vi "Fetch Waveform.vi"(8 "error in (no error)":errorcluster, 9 "Timeout (10000 ms)":u32=10000, 10 "Channel (1: Channel 1)":u16(ring)=1 items=["Channel 1"=1, "Channel 2"=2, "Channel 3"=3, "Channel 4"=4], 11 "VISA resource name":refnum<visa-resource-name>) -> (0 "error out":errorcluster, 2 "Waveform Data":waveform(dbl)(graph), 3 "VISA resource name out":refnum<visa-resource-name>)   [LabVIEW 2023, in "RIGOL DS1054Z Driver.lvlib"]
doc: "Returns the waveform the oscilloscope acquired for the specified channel. The waveform is from an acquisition that you initiate prior to calling this VI.\n\n<B>Note:</B>\n Use this VI only with other low-level VIs."
uses:
  <instrlib>/RIGOL-DS1054Z-LabVIEW/RIGOL DS1054Z Driver.lvlib
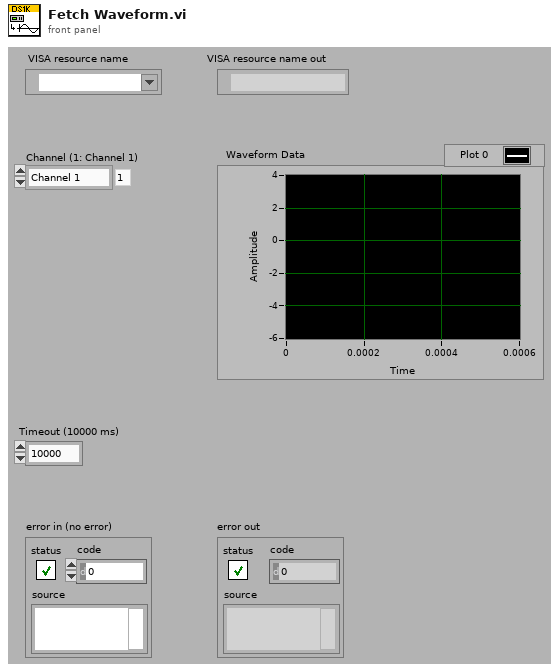
[diagram p1: front panel]
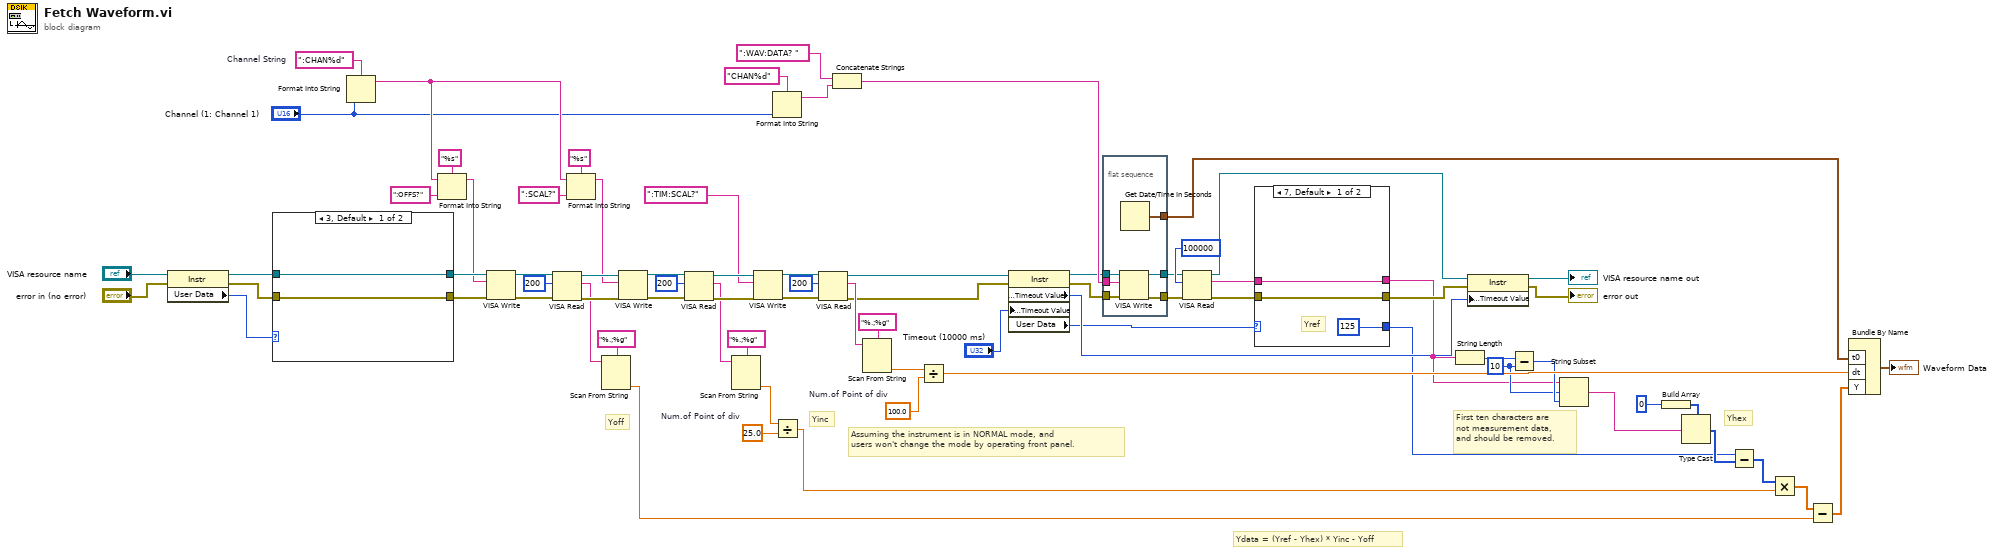
[diagram p0: block diagram]
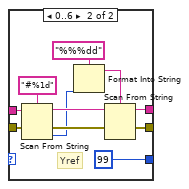
[diagram p2: hidden frame]
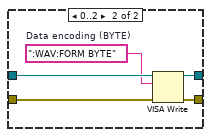
[diagram p3: hidden frame]
diagram:
  w6 = ":CHAN%d"  # Channel String
  w9 = 10 ("y")
  w21 = 100.0  # Num.of Point of div
  w30 = 25.0  # Num.of Point of div
  # "Assuming the instrument is in NORMAL mode, and \nusers won't change the mode by operating front panel."
  # "First ten characters are\nnot measurement data, \nand should be removed."
  # "Yoff"
  # "Yinc"
  # "Yhex"
  # "Ydata = (Yref - Yhex) * Yinc - Yoff"
  n1 = property class="Instr"(reference="VISA resource name", error in="error in (no error)") -> (reference out=w60:refnum<visa-resource-name>, error out=w58:errorcluster, "User Data"=w39:u32)
  n2 = case shown="3, Default" w39 {
    tunnel: [w79 w84] -> w57
    tunnel: [w78 w83] -> w56
    tunnel: w60 -> [w79 w82]
    tunnel: w58 -> [w78 w81]
    frame 3, Default {
    }
    frame 0..2 {
      w80 = ":WAV:FORM BYTE"  # Data encoding (BYTE)
      n3 = VISA Write(VISA resource name=w82, write buffer=w80, error in (no error)=w81) -> (VISA resource name out=w84:refnum<visa-resource-name>, error out=w83:errorcluster)  [unwired: 1 out]
    }
  }
  n4 = Format Into String(format string=w6, "Channel (1: Channel 1)") -> (resulting string=w5:string)  [unwired: 2 in, 1 out]
  n5 = Format Into String(format string="%s" ("格式字符串"), initial string=w5, ":OFFS?") -> (resulting string=w36:string)  [unwired: 1 in, 1 out]
  n6 = VISA Write(VISA resource name=w57, write buffer=w36, error in (no error)=w56) -> (VISA resource name out=w55:refnum<visa-resource-name>, error out=w54:errorcluster)  [unwired: 1 out]
  n7 = VISA Read(VISA resource name=w55, byte count=u32 200, error in (no error)=w54) -> (VISA resource name out=w47:refnum<visa-resource-name>, read buffer=w38:string, error out=w46:errorcluster)  [unwired: 1 out]
  n8 = Format Into String(format string="%s" ("格式字符串"), initial string=w5, ":SCAL?") -> (resulting string=w35:string)  [unwired: 1 in, 1 out]
  n9 = Scan From String(format string="%.;%g", input string=w38) -> (output 1=w24:dbl)  [unwired: 2 in, 4 out]
  n10 = VISA Write(VISA resource name=w47, write buffer=w35, error in (no error)=w46) -> (VISA resource name out=w52:refnum<visa-resource-name>, error out=w53:errorcluster)  [unwired: 1 out]
  n11 = VISA Read(VISA resource name=w52, byte count=u32 200, error in (no error)=w53) -> (VISA resource name out=w43:refnum<visa-resource-name>, read buffer=w31:string, error out=w42:errorcluster)  [unwired: 1 out]
  n12 = Scan From String(format string="%.;%g", input string=w31) -> (output 1=w28:dbl)  [unwired: 2 in, 4 out]
  n13 = VISA Write(VISA resource name=w43, write buffer=":TIM:SCAL?", error in (no error)=w42) -> (VISA resource name out=w49:refnum<visa-resource-name>, error out=w48:errorcluster)  [unwired: 1 out]
  n14 = Format Into String(format string="CHAN%d" ("Channel String"), "Channel (1: Channel 1)") -> (resulting string=w3:string)  [unwired: 2 in, 1 out]
  n15 = Divide(x=w28, y=w30) -> (x/y=w26:dbl)
  n16 = VISA Read(VISA resource name=w49, byte count=u32 200, error in (no error)=w48) -> (VISA resource name out=w14:refnum<visa-resource-name>, read buffer=w33:string, error out=w17:errorcluster)  [unwired: 1 out]
  n17 = Concatenate Strings(":WAV:DATA? " ("write buffer"), w3) -> (w62:string)
  n18 = Scan From String(format string="%.;%g", input string=w33) -> (output 1=w22:dbl)  [unwired: 2 in, 4 out]
  n19 = Divide(x=w22, y=w21) -> (x/y=w20:dbl)
  n20 = property class="Instr"(reference=w14, error in=w17, "General Settings:Timeout Value"="Timeout (10000 ms)") -> (reference out=w13:refnum<visa-resource-name>, error out=w16:errorcluster, "General Settings:Timeout Value"=w67:u32, "User Data"=w19:u32)
  n21 = flat-sequence {
    tunnel: w62 -> [w90]
    tunnel: w16 -> [w89]
    tunnel: [w88] -> w15
    tunnel: w13 -> [w87]
    tunnel: [w86] -> w12
    tunnel: [w85] -> w1
    frame #0 {
      n22 = VISA Write(VISA resource name=w87, write buffer=w90, error in (no error)=w89) -> (VISA resource name out=w86:refnum<visa-resource-name>, error out=w88:errorcluster)  [unwired: 1 out]
      n23 = Get Date/Time In Seconds() -> (seconds since 1Jan1904=w85:timestamp)
    }
  }
  n24 = VISA Read(VISA resource name=w12, byte count=u32 100000, error in (no error)=w15) -> (VISA resource name out=w71:refnum<visa-resource-name>, read buffer=w66:string, error out=w64:errorcluster)  [unwired: 1 out]
  n25 = case shown="7, Default" w19 {
    tunnel: [w93 w104] -> w8
    tunnel: [w92 w103] -> w70
    tunnel: w66 -> [w93 w96]
    tunnel: w64 -> [w92 w95]
    tunnel: [i16 125 ("t") i16 99 ("f")] -> w18
    frame 7, Default {
      # "Yref"
    }
    frame 0..6 {
      # "Yref"
      n26 = Scan From String(format string="#%1d", input string=w96, error in=w95) -> (remaining string=w100:string, error out=w98:errorcluster, output 1=w97:i32)  [unwired: 1 in, 2 out]
      n27 = Format Into String(format string="%%%dd", w97) -> (resulting string=w99:string)  [unwired: 2 in, 1 out]
      n28 = Scan From String(format string=w99, input string=w100, error in=w98) -> (remaining string=w104:string, error out=w103:errorcluster)  [unwired: 1 in, 3 out]
    }
  }
  n29 = String Length(string=w8) -> (length=w11:i32)
  n30 = property class="Instr"(reference=w71, error in=w70, "General Settings:Timeout Value"=w67) -> (reference out=→"VISA resource name out":refnum<visa-resource-name>, error out=→"error out":errorcluster)
  n31 = Subtract(x=w11, y=w9) -> (x-y=w10:i32)
  n32 = String Subset(string=w8, offset (0)=w9, length (rest)=w10) -> (substring=w7:string)
  n33 = Build Array(u8 0) -> (w75:u8[])
  n34 = Type Cast(type=w75, x=w7) -> (*(type *) &x=w29:u8[])
  n35 = Subtract(x=w18, y=w29) -> (x-y=w27:i16[])
  n36 = Multiply(x=w27, y=w26) -> (x*y=w25:dbl[])
  n37 = Subtract(x=w25, y=w24) -> (x-y=w23:dbl[])
  n38 = Bundle By Name("t0"=w1, "dt"=w20, "Y"=w23) -> (→"Waveform Data":waveform(dbl))  [unwired: 1 out]
